vi "Main IU.vi"() -> ()   [LabVIEW 2019]
uses:
  <vilib>/Analysis/baseanly.llb/Mean (DBL).vi
  <vilib>/Analysis/NI_AALBase.lvlib
panel:
  out "Motor Codo":waveform(dbl)[](graph)
  in  "Stop UI and RT":bool
  in  "Stop UI":bool
  in  "Controladores e Indicadores":enum32{"TCD || TCI", "Guardar Datos"}(tab)
  in  "px":dbl
  in  "py":dbl
  in  "Codo":bool
  in  "Hombro":bool
  in  "codo arriba":bool
  in  "enviar coordenadas":bool
  in  "enviar trayectoria":bool
  in  "tiempo final":dbl
  out "Fuera del espacio de trabajo":bool[](array[boolean])
  out "Posición en X":dbl[](array[numeric])
  out "Posición en Y":dbl[](array[numeric])
  in  "Filename":path=path "test.lvm"
  in  "Record Button":bool
  out "Saving Data":bool
  in  "Selector":bool
  out "Motor Hombro":waveform(dbl)[](graph)
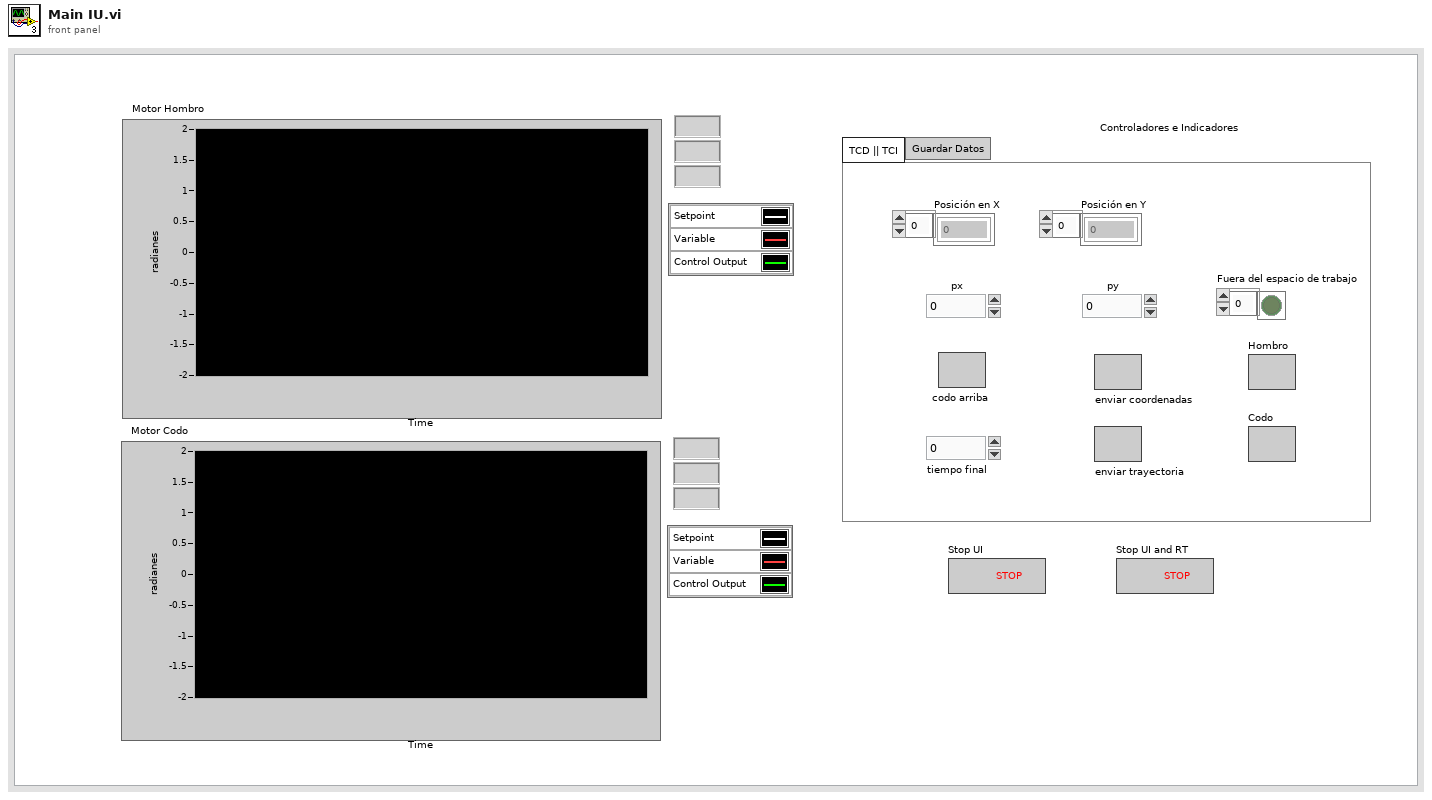
[diagram p1: front panel]
types:
  T1 = cluster{"seconds since 1Jan1904":timestamp, dbl, dbl, "uk":dbl, dbl, "setpoint (rads)":dbl, "encoder (rads)":dbl, "uk":dbl, "error":dbl, "px":dbl, "py":dbl, "fueraEspacioDeTrabajo":bool}
  T2 = cluster{"seconds since 1Jan1904":timestamp, dbl, dbl, "uk":dbl, dbl, "setpoint (rads)":dbl, "encoder (rads)":dbl, "uk":dbl, "error":dbl, "px":dbl, "py":dbl, "fueraEspacioDeTrabajo":bool}[]
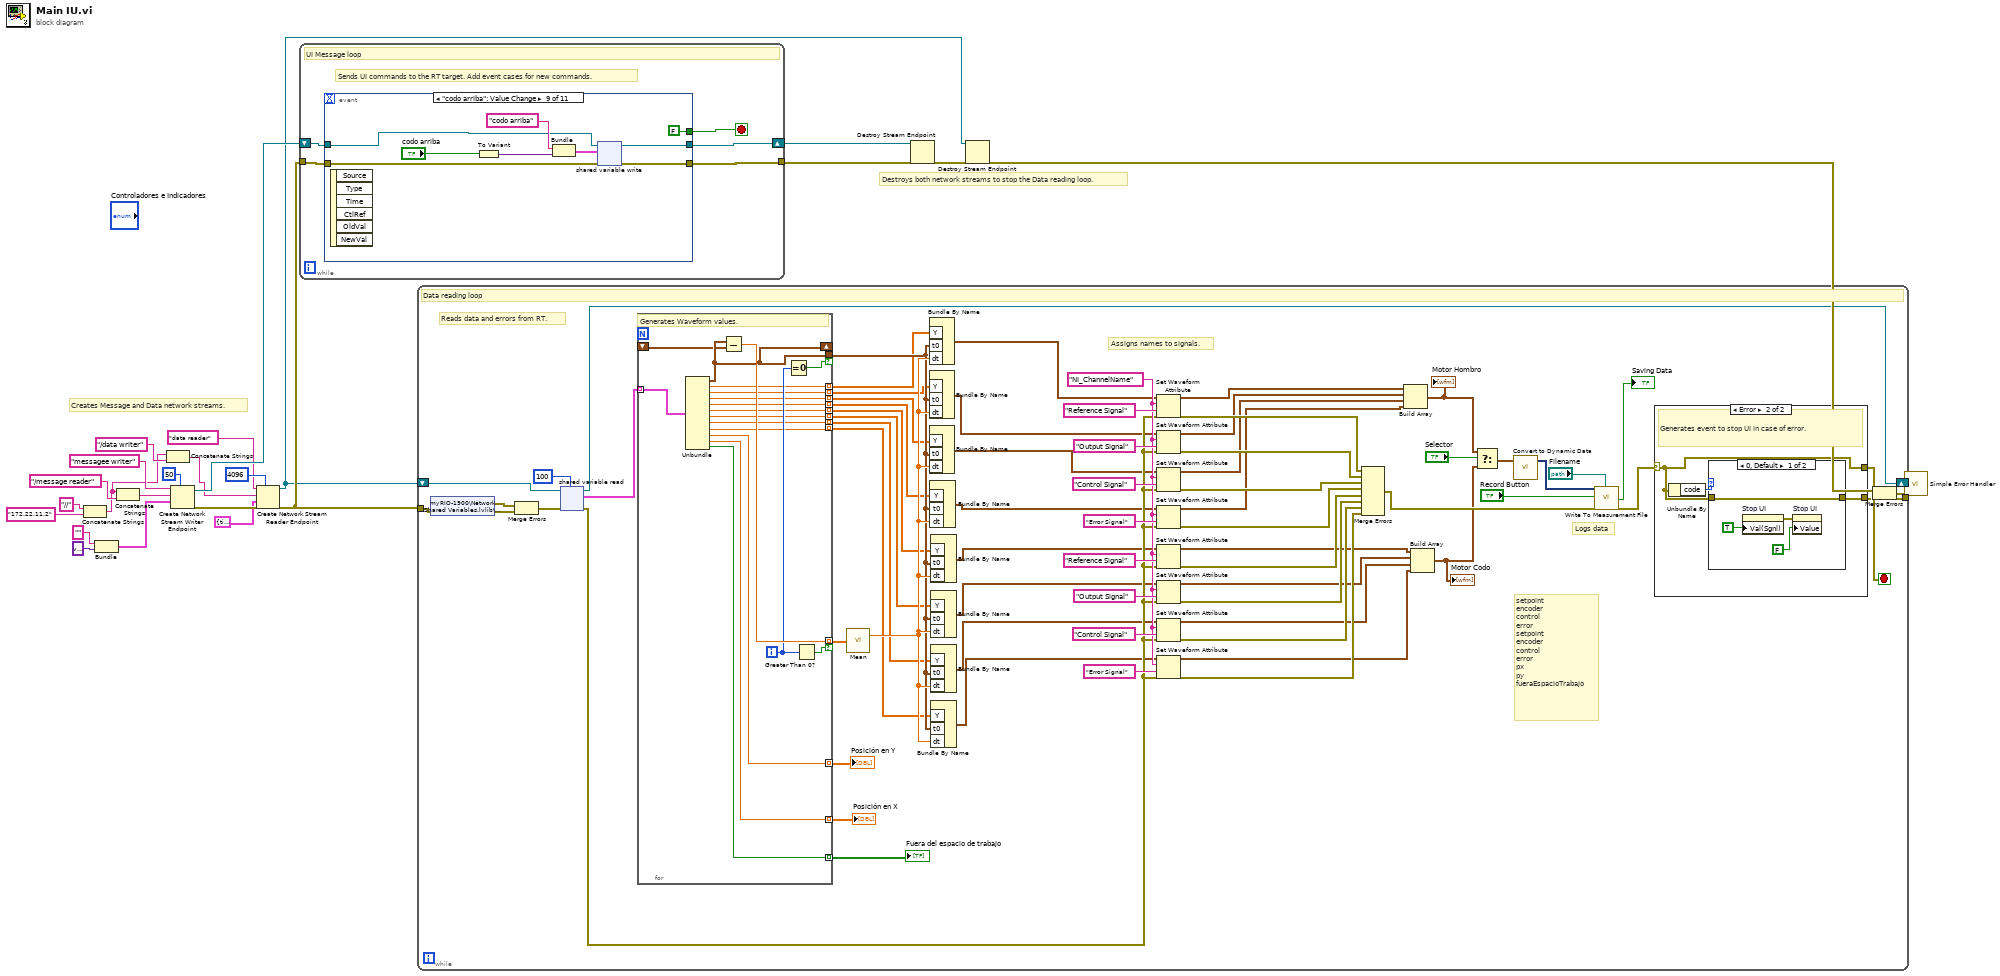
[diagram p0: block diagram]
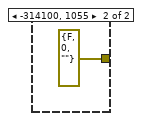
[diagram p3: hidden frame]
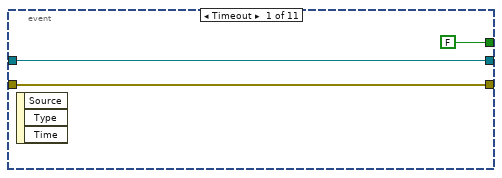
[diagram p4: hidden frame]
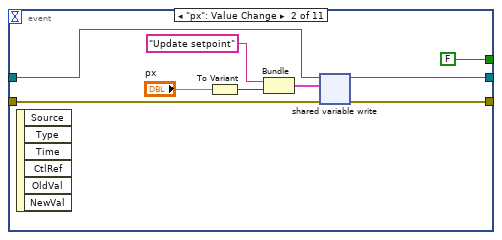
[diagram p5: hidden frame]
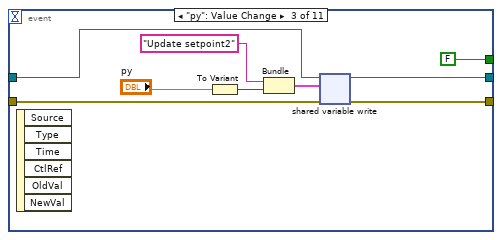
[diagram p6: hidden frame]
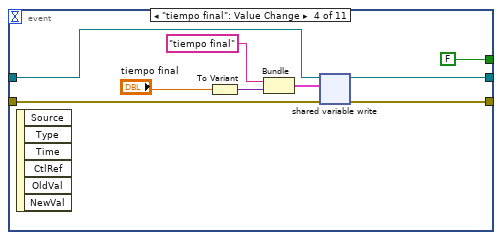
[diagram p7: hidden frame]
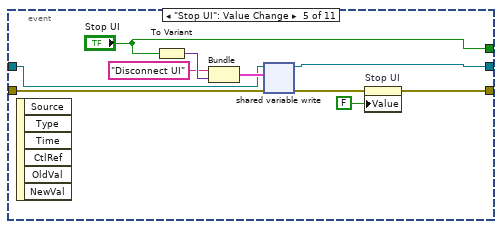
[diagram p8: hidden frame]
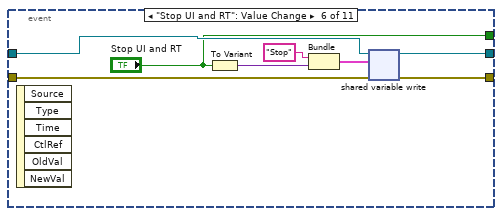
[diagram p9: hidden frame]
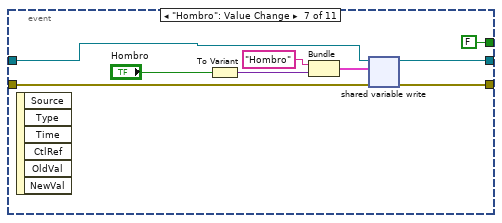
[diagram p10: hidden frame]
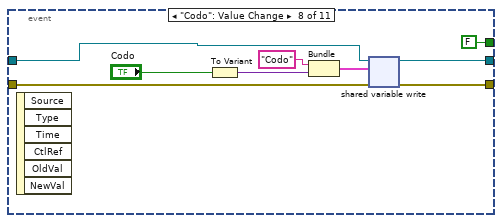
[diagram p11: hidden frame]
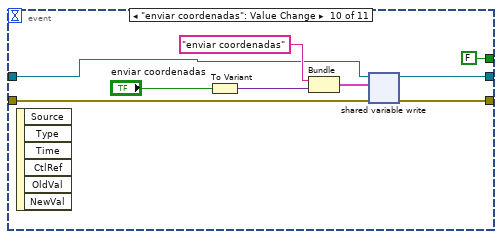
[diagram p12: hidden frame]
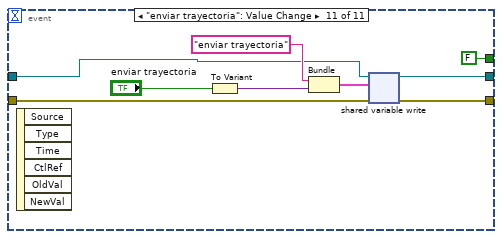
[diagram p13: hidden frame]
diagram:
  # "Destroys both network streams to stop the Data reading loop."
  # "Creates Message and Data network streams."
  n1 = Concatenate Strings("//", "172.22.11.2" ("myRIO IP")) -> (w2:string)
  n2 = Bundle("", variant) -> (w25:cluster{string, variant})  [unwired: 1 in]
  n3 = Concatenate Strings(w2, "/message reader") -> (w3:string)
  n4 = Concatenate Strings(w2, "/data writer") -> (w16:string)
  n5 = Create Network Stream Writer Endpoint(7:50 ("writer buffer size"), 9:w25, 10:w3, 11:"messagee writer" ("writer name")) -> (0:w13:errorcluster, 3:w19:refnum<k21>)  [unwired: 3 in]
  n6 = Create Network Stream Reader Endpoint(7:4096 ("reader buffer size"), 8:w13, 9:T1 {"seconds since 1Jan1904"=timestamp(0 s since 1904-01-01), 0.0, 0.0, "uk"=0.0, 0.0, "setpoint (rads)"=0.0, "encoder (rads)"=0.0, "uk"=0.0, "error"=0.0, "px"=0.0, "py"=0.0, "fueraEspacioDeTrabajo"=FALSE} ("output cluster"), 10:w16, 11:"data reader" ("reader name")) -> (0:w12:errorcluster, 3:w6:refnum<k21>)  [unwired: 2 in]
  n7 = while {
    tunnel: w12 -> [w29]
    shift-right: [w28] -> w8
    shift-left: w19 -> [w30]
    tunnel: [w27] -> w9
    stop <- w26 stop-if-true
    # "Sends UI commands to the RT target. Add event cases for new commands."
    # "UI Message loop"
    n8 = event shown="[8] \"codo arriba\": Value Change" {
      selector: _ -> [_ _ _ _ _ _ _ _ _ _ _]
      dyn-events: _ -> [_ _ _ _ _ _ _ _ _ _ _]
      timeout: _ -> [_ _ _ _ _ _ _ _ _ _ _]
      tunnel: w30 -> [w33 w42 w51 w60 w67 w72 w81 w90 w99 w108 w117]
      tunnel: w29 -> [w31 w41 w50 w59 w63 w75 w84 w93 w102 w111 w120]
      tunnel: [w33 w36 w46 w55 w66 w73 w82 w91 w100 w109 w118] -> w28
      tunnel: [w31 w35 w45 w54 w61 w74 w83 w92 w101 w110 w119] -> w27
      tunnel: [FALSE ("Stop UI and RT") FALSE ("Stop UI and RT") FALSE ("Stop UI and RT") FALSE ("Stop UI and RT") "Stop UI" "Stop UI and RT" FALSE ("Codo") FALSE ("Codo") FALSE ("Codo") FALSE ("Codo") FALSE ("Codo")] -> w26
      event Timeout {
        n9 = event-data() -> ()  [unwired: 1 in, 3 out]
      }
      event "px": Value Change {
        n10 = event-data() -> ()  [unwired: 1 in, 6 out]
        n11 = To Variant(anything="px") -> (Variant=w40:variant)
        n12 = Bundle("writer name"="Update setpoint", "Variant"=w40) -> (w37:cluster{"writer name":string, "Variant":variant})  [unwired: 1 in]
        n13 = shared-variable-write(w42, w41, w37) -> (w36:refnum<k21>, w35:errorcluster)  [unwired: 1 in, 1 out]
      }
      event "py": Value Change {
        n14 = event-data() -> ()  [unwired: 1 in, 6 out]
        n15 = To Variant(anything="py") -> (Variant=w49:variant)
        n16 = Bundle("writer name"="Update setpoint2", "Variant"=w49) -> (w47:cluster{"writer name":string, "Variant":variant})  [unwired: 1 in]
        n17 = shared-variable-write(w51, w50, w47) -> (w46:refnum<k21>, w45:errorcluster)  [unwired: 1 in, 1 out]
      }
      event "tiempo final": Value Change {
        n18 = event-data() -> ()  [unwired: 1 in, 6 out]
        n19 = To Variant(anything="tiempo final") -> (Variant=w58:variant)
        n20 = Bundle("writer name"="tiempo final", "Variant"=w58) -> (w56:cluster{"writer name":string, "Variant":variant})  [unwired: 1 in]
        n21 = shared-variable-write(w60, w59, w56) -> (w55:refnum<k21>, w54:errorcluster)  [unwired: 1 in, 1 out]
      }
      event "Stop UI": Value Change {
        n22 = event-data() -> ()  [unwired: 1 in, 6 out]
        n23 = To Variant(anything="Stop UI") -> (Variant=w70:variant)
        n24 = Bundle("writer name"="Disconnect UI", "Variant"=w70) -> (w69:cluster{"writer name":string, "Variant":variant})  [unwired: 1 in]
        n25 = shared-variable-write(w67, w63, w69) -> (w66:refnum<k21>, w62:errorcluster)  [unwired: 1 in, 1 out]
        n26 = property on="Stop UI" class="Bool (strict)"(error in=w62, "Value"=FALSE ("Stop UI and RT")) -> (error out=w61:errorcluster)  [unwired: 1 in, 1 out]
      }
      event "Stop UI and RT": Value Change {
        n27 = event-data() -> ()  [unwired: 1 in, 6 out]
        n28 = To Variant(anything="Stop UI and RT") -> (Variant=w78:variant)
        n29 = Bundle("writer name"="Stop", "Variant"=w78) -> (w77:cluster{"writer name":string, "Variant":variant})  [unwired: 1 in]
        n30 = shared-variable-write(w72, w75, w77) -> (w73:refnum<k21>, w74:errorcluster)  [unwired: 1 in, 1 out]
      }
      event "Hombro": Value Change {
        n31 = event-data() -> ()  [unwired: 1 in, 6 out]
        n32 = To Variant(anything="Hombro") -> (Variant=w87:variant)
        n33 = Bundle("writer name"="Hombro", "Variant"=w87) -> (w86:cluster{"writer name":string, "Variant":variant})  [unwired: 1 in]
        n34 = shared-variable-write(w81, w84, w86) -> (w82:refnum<k21>, w83:errorcluster)  [unwired: 1 in, 1 out]
      }
      event "Codo": Value Change {
        n35 = event-data() -> ()  [unwired: 1 in, 6 out]
        n36 = To Variant(anything="Codo") -> (Variant=w96:variant)
        n37 = Bundle("writer name"="Codo", "Variant"=w96) -> (w95:cluster{"writer name":string, "Variant":variant})  [unwired: 1 in]
        n38 = shared-variable-write(w90, w93, w95) -> (w91:refnum<k21>, w92:errorcluster)  [unwired: 1 in, 1 out]
      }
      event "codo arriba": Value Change {
        n39 = event-data() -> ()  [unwired: 1 in, 6 out]
        n40 = To Variant(anything="codo arriba") -> (Variant=w105:variant)
        n41 = Bundle("writer name"="codo arriba", "Variant"=w105) -> (w104:cluster{"writer name":string, "Variant":variant})  [unwired: 1 in]
        n42 = shared-variable-write(w99, w102, w104) -> (w100:refnum<k21>, w101:errorcluster)  [unwired: 1 in, 1 out]
      }
      event "enviar coordenadas": Value Change {
        n43 = event-data() -> ()  [unwired: 1 in, 6 out]
        n44 = To Variant(anything="enviar coordenadas") -> (Variant=w114:variant)
        n45 = Bundle("writer name"="enviar coordenadas", "Variant"=w114) -> (w113:cluster{"writer name":string, "Variant":variant})  [unwired: 1 in]
        n46 = shared-variable-write(w108, w111, w113) -> (w109:refnum<k21>, w110:errorcluster)  [unwired: 1 in, 1 out]
      }
      event "enviar trayectoria": Value Change {
        n47 = event-data() -> ()  [unwired: 1 in, 6 out]
        n48 = To Variant(anything="enviar trayectoria") -> (Variant=w123:variant)
        n49 = Bundle("writer name"="enviar trayectoria", "Variant"=w123) -> (w122:cluster{"writer name":string, "Variant":variant})  [unwired: 1 in]
        n50 = shared-variable-write(w117, w120, w122) -> (w118:refnum<k21>, w119:errorcluster)  [unwired: 1 in, 1 out]
      }
    }
  }
  n51 = while {
    tunnel: w12 -> [w178]
    shift-right: [w188] -> _
    shift-left: w6 -> [w191]
    tunnel: [w177] -> w10
    stop <- w176 stop-if-true
    w167 = "NI_ChannelName" ("name")
    # "setpoint\nencoder\ncontrol\nerror\nsetpoint\nencoder\ncontrol\nerror\npx\npy\nfueraEspacioTrabajo"
    # "Logs data"
    # "Assigns names to signals."
    # "Reads data and errors from RT."
    # "Data reading loop"
    n52 = shared-variable "myRIO-1900\\Network Shared Variables.lvlib\\error IO"(error in=w178) -> (w181:errorcluster, error out=w180:errorcluster)
    n53 = Merge Errors(w181, w180) -> (w179:errorcluster)
    n54 = shared-variable-read(w191, w179, 100 ("# elements")) -> (w188:refnum<k21>, w158:errorcluster, w189:T2)  [unwired: 1 in, 1 out]
    n55 = for {
      tunnel: w189 -> [w218] mode=indexing
      tunnel: [w213] -> w155 if=w215
      shift-right: [w213] -> _
      shift-left: _ -> [w212]
      tunnel: [w217] -> w182 mode=indexing if=w214
      tunnel: [w211] -> w154 mode=indexing
      tunnel: [w210] -> w153 mode=indexing
      tunnel: [w209] -> w152 mode=indexing
      tunnel: [w208] -> w151 mode=indexing
      tunnel: [w207] -> w150 mode=indexing
      tunnel: [w206] -> w149 mode=indexing
      tunnel: [w205] -> w148 mode=indexing
      tunnel: [w204] -> w147 mode=indexing
      tunnel: [w203] -> w126 mode=indexing
      tunnel: [w202] -> w125 mode=indexing
      tunnel: [w201] -> w124 mode=indexing
      i -> [w216]
      # "Generates Waveform values."
      n56 = Unbundle(w218) -> ("seconds since 1Jan1904"=w213:timestamp, w211:dbl, w210:dbl, "uk"=w209:dbl, w208:dbl, "setpoint (rads)"=w207:dbl, "encoder (rads)"=w206:dbl, "uk"=w205:dbl, "error"=w204:dbl, "px"=w203:dbl, "py"=w202:dbl, "fueraEspacioDeTrabajo"=w201:bool)
      n57 = Subtract(x=w213, y=w212) -> (x-y=w217:dbl)
      n58 = Equal To 0?(x=w216) -> (x = 0?=w215:bool)
      n59 = Greater Than 0?(x=w216) -> (x > 0?=w214:bool)
    }
    "Posición en Y" <- w126
    "Posición en X" <- w125
    "Fuera del espacio de trabajo" <- w124
    n60 = call-poly <vilib>:"Mean.vi"("X"=w182) -> ("mean"=w156:dbl)  [unwired: 1 out]
    n61 = Bundle By Name("Y"=w154, "t0"=w155, "dt"=w156) -> (w146:waveform(dbl))  [unwired: 1 in]
    n62 = Bundle By Name("Y"=w153, "t0"=w155, "dt"=w156) -> (w145:waveform(dbl))  [unwired: 1 in]
    n63 = Bundle By Name("Y"=w152, "t0"=w155, "dt"=w156) -> (w144:waveform(dbl))  [unwired: 1 in]
    n64 = Bundle By Name("Y"=w151, "t0"=w155, "dt"=w156) -> (w143:waveform(dbl))  [unwired: 1 in]
    n65 = Bundle By Name("Y"=w150, "t0"=w155, "dt"=w156) -> (w142:waveform(dbl))  [unwired: 1 in]
    n66 = Bundle By Name("Y"=w149, "t0"=w155, "dt"=w156) -> (w141:waveform(dbl))  [unwired: 1 in]
    n67 = Bundle By Name("Y"=w148, "t0"=w155, "dt"=w156) -> (w140:waveform(dbl))  [unwired: 1 in]
    n68 = Bundle By Name("Y"=w147, "t0"=w155, "dt"=w156) -> (w139:waveform(dbl))  [unwired: 1 in]
    n69 = Set Waveform Attribute(4:w158, 5:"Reference Signal" ("name"), 6:w167, 7:w146) -> (0:w166:errorcluster, 3:w138:waveform(dbl))  [unwired: 1 out]
    n70 = Set Waveform Attribute(4:w158, 5:"Output Signal" ("name"), 6:w167, 7:w145) -> (0:w165:errorcluster, 3:w137:waveform(dbl))  [unwired: 1 out]
    n71 = Set Waveform Attribute(4:w158, 5:"Control Signal" ("name"), 6:w167, 7:w144) -> (0:w164:errorcluster, 3:w136:waveform(dbl))  [unwired: 1 out]
    n72 = Set Waveform Attribute(4:w158, 5:"Error Signal" ("name"), 6:w167, 7:w143) -> (0:w163:errorcluster, 3:w135:waveform(dbl))  [unwired: 1 out]
    n73 = Set Waveform Attribute(4:w158, 5:"Reference Signal" ("name"), 6:w167, 7:w142) -> (0:w162:errorcluster, 3:w134:waveform(dbl))  [unwired: 1 out]
    n74 = Set Waveform Attribute(4:w158, 5:"Output Signal" ("name"), 6:w167, 7:w141) -> (0:w161:errorcluster, 3:w133:waveform(dbl))  [unwired: 1 out]
    n75 = Set Waveform Attribute(4:w158, 5:"Control Signal" ("name"), 6:w167, 7:w140) -> (0:w160:errorcluster, 3:w132:waveform(dbl))  [unwired: 1 out]
    n76 = Set Waveform Attribute(4:w158, 5:"Error Signal" ("name"), 6:w167, 7:w139) -> (0:w159:errorcluster, 3:w131:waveform(dbl))  [unwired: 1 out]
    n77 = Merge Errors(w166, w165, w164, w163, w162, w161, w160, w159) -> (w157:errorcluster)
    n78 = Build Array(w138, w137, w136, w135) -> (w129:waveform(dbl)[])
    "Motor Hombro" <- w129
    n79 = Build Array(w134, w133, w132, w131) -> (w128:waveform(dbl)[])
    "Motor Codo" <- w128
    n80 = Select(t=w129, s="Selector", f=w128) -> (s? t:f=w130:waveform(dbl)[])
    n81 = call "Convert to Dynamic Data"("Array of Waveforms"=w130) -> ("Dynamic Data Type"=w187:dynamicdata)  [unwired: 3 in]
    n82 = call "Write To Measurement File"("Signals"=w187, "Enable"="Record Button", "error in (no error)"=w157, "Filename"="Filename") -> ("Saving Data"=→"Saving Data":bool, "error out"=w183:errorcluster)  [unwired: 13 in, 1 out]
    n83 = case shown="Error" w183 {
      selector: w183 -> [w192 w193]
      tunnel: [w192 w194] -> w177
      tunnel: [w192 w193] -> w176
      frame No Error {
        # "No action required."
      }
      frame Error {
        # "Generates event to stop UI in case of error."
        n84 = Unbundle By Name(w193) -> ("code"=w195:i32)
        n85 = case shown="0, Default" w195 {
          tunnel: [w198 errorcluster {"status"=FALSE, "code"=0, "source"=""} ("error IO")] -> w194
          tunnel: w193 -> [w198 _]
          frame 0, Default {
            n86 = property on="Stop UI" class="Bool (strict)"("Val(Sgnl)"=TRUE ("Stop UI and RT")) -> (error out=w197:errorcluster)  [unwired: 2 in, 1 out]
            n87 = property on="Stop UI" class="Bool (strict)"(error in=w197, "Value"=FALSE ("Stop UI")) -> ()  [unwired: 1 in, 2 out]
          }
          frame -314100, 1055 {
          }
        }
      }
    }
  }
  n88 = Destroy Stream Endpoint(8:w9, 11:w8) -> (0:w7:errorcluster)
  n89 = Destroy Stream Endpoint(8:w7, 11:w6) -> (0:w5:errorcluster)
  n90 = Merge Errors(w5, w10) -> (w11:errorcluster)
  n91 = call <vilib>:"Simple Error Handler.vi"("error in (no error)"=w11) -> ()  [unwired: 4 in, 5 out]
